vi "PosCtrl_Execute.vi"(5 "PosCtrl_Config_Params":T1={"Slope"=0.0, "Offset"=0.0, "Error Deadband"=0.0, "At Reference Count"=13, "Negate Output"=FALSE, "Max Allowd Position"=9e+30, "Min Allowd Position"=-9e+30}, 7 "MaxOutput":dbl, 8 "Rev Limit Switch":bool, 9 "Fwd Limit Switch":bool, 10 "CurrentPosition":dbl, 11 "TargetPosition":dbl) -> (1 "OnTarget":bool, 2 "PositionError":dbl, 3 "Output":dbl)   [LabVIEW 2019, in "Trajectory_Library.lvlib"]
doc: "This VI calculates closed loop position control output (CO), provided the Setpoint (SP), and Process Variable (PV). It incorporates a position deadband. It also incorporates output slowdown as the desired position is approached."
uses:
  TypeDef/PosCtrl_Tuning_Type.ctl
  Trajectory_Library.lvlib
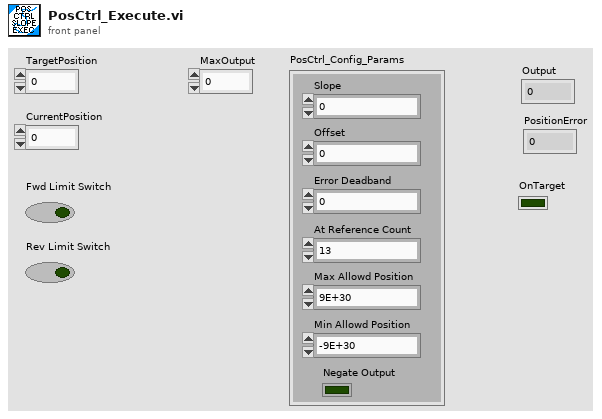
[diagram p1: front panel]
types:
  T1 = typedef "Trajectory_Library.lvlib/PosCtrl_Tuning_Type.ctl" = cluster{"Slope":dbl, "Offset":dbl, "Error Deadband":dbl, "At Reference Count":i32, "Negate Output":bool, "Max Allowd Position":dbl, "Min Allowd Position":dbl}
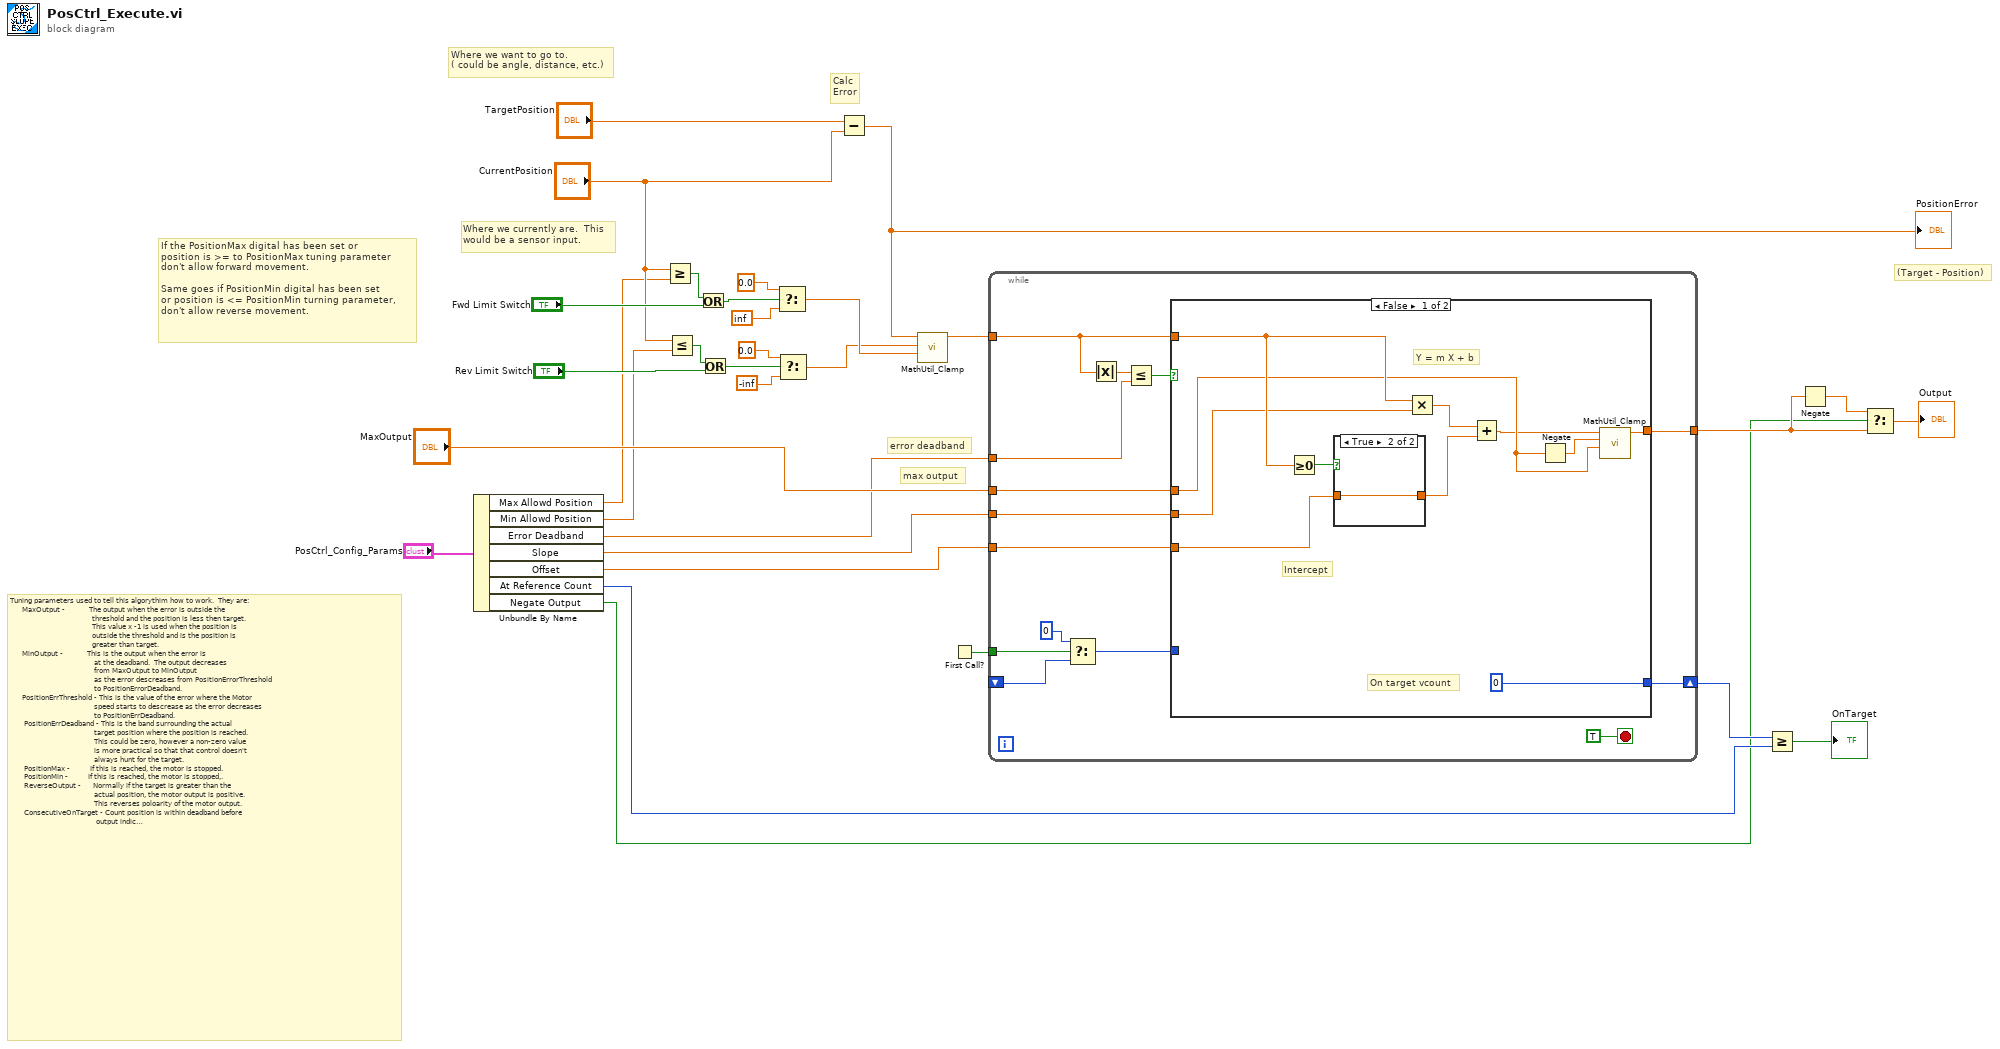
[diagram p0: block diagram]
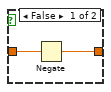
[diagram p2: hidden frame]
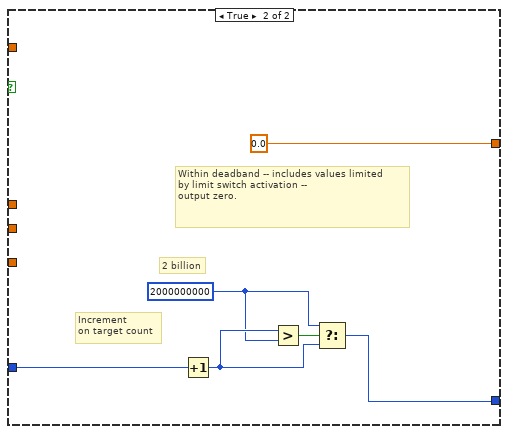
[diagram p3: hidden frame]
diagram:
  # "error deadband"
  # "max output"
  # "(Target - Position)"
  # "Calc\nError"
  # "If the PositionMax digital has been set or\nposition is >= to PositionMax tuning parameter\ndon't allow forward movement.\n\nSame goes if PositionMin digital has been set\nor position is <= PositionMin turning parameter, \ndon't allow reverse movement."
  # "Tuning parameters used to tell this algorythim how to work.  They are:\n      MaxOutput -            The output when the error is outside the \n                                         threshold and the position is less then target.\n                                         This value x -1 is used when the position is\n                                         outside the threshold and is the position is\n                                         greater than target.\n      MinOutput -            This is the output when the error is\n                                          at the deadband.  The output decreases\n                                          from MaxOutput to MinOutput\n                                          as the error descreases from PositionErrorThreshold\n                                          to PositionErrorDeadband.\n      PositionErrThreshold - This is the value of the error where the Motor\n                                          speed starts to descrease as the error decreases\n                                          to PositionErrDeadband.\n       PositionErrDeadband - This is the band surrounding the actual \n                                          target position where the position is reached.\n                                          This could be zero, however a non-zero value\n                                          is more practical so that that control doesn't\n                                          always hunt for the target.\n       PositionMax -          If this is reached, the motor is stopped.\n       PositionMin -          If this is reached, the motor is stopped,.\n       ReverseOutput -      Normally if the target is greater than the \n                                          actual position, the motor output is positive.\n                                          This reverses poloarity of the motor output.\n       ConsecutiveOnTarget - Count position is within deadband before\n                                           output indicates position goal has been\n                                           reached."
  # "Where we currently are.  This \nwould be a sensor input."
  # "Where we want to go to.\n( could be angle, distance, etc.)"
  n1 = Unbundle By Name("PosCtrl_Config_Params") -> ("Max Allowd Position"=w11:dbl, "Min Allowd Position"=w10:dbl, "Error Deadband"=w21:dbl, "Slope"=w20:dbl, "Offset"=w19:dbl, "At Reference Count"=w9:i32, "Negate Output"=w5:bool)
  n2 = Greater Or Equal?(x="CurrentPosition", y=w11) -> (x >= y?=w13:bool)
  n3 = Less Or Equal?(x="CurrentPosition", y=w10) -> (x <= y?=w14:bool)
  n4 = Or(x=w13, y="Fwd Limit Switch") -> (x .or. y?=w18:bool)
  n5 = Or(x=w14, y="Rev Limit Switch") -> (x .or. y?=w17:bool)
  n6 = Select(t=0.0, s=w18, f=inf) -> (s? t:f=w3:dbl)
  n7 = Select(t=0.0, s=w17, f=-inf) -> (s? t:f=w2:dbl)
  n8 = Subtract(x="TargetPosition", y="CurrentPosition") -> (x-y=w4:dbl)
  "PositionError" <- w4
  n9 = call "MathUtil_Clamp.vi"("High Limit"=w3, "Low Limit"=w2, "Value"=w4) -> ("Result"=w1:dbl)  [unwired: 8 in]
  n10 = First Call?() -> (First Call?: T/F=w26:bool)
  n11 = while {
    tunnel: w1 -> [w41]
    tunnel: w21 -> [w34]
    tunnel: [w42] -> w6
    tunnel: "MaxOutput" -> [w40]
    shift-right: [w39] -> w24
    shift-left: _ -> [w37]
    tunnel: w26 -> [w38]
    tunnel: w19 -> [w33]
    tunnel: w20 -> [w32]
    stop <- TRUE stop-if-true
    n12 = Select(t=0, s=w38, f=w37) -> (s? t:f=w36:i32)
    n13 = Absolute Value(x=w41) -> (abs(x)=w45:dbl)
    n14 = Less Or Equal?(x=w45, y=w34) -> (x <= y?=w43:bool)
    n15 = case shown="False" w43 {
      tunnel: [w46 0.0] -> w42
      tunnel: w41 -> [w56 _]
      tunnel: w40 -> [w48 _]
      tunnel: [0 w61] -> w39
      tunnel: w36 -> [_ w64]
      tunnel: w33 -> [w51 _]
      tunnel: w32 -> [w50 _]
      frame False {
        # "Y = m X + b"
        # "Intercept"
        # "On target vcount"
        n16 = Greater Or Equal To 0?(x=w56) -> (x >= 0?=w54:bool)
        n17 = case shown="True" w54 {
          tunnel: w51 -> [w58 w59]
          tunnel: [w57 w59] -> w52
          frame False {
            n18 = Negate(x=w58) -> (-x=w57:dbl)
          }
          frame True {
          }
        }
        n19 = Multiply(x=w56, y=w50) -> (x*y=w53:dbl)
        n20 = Add(x=w53, y=w52) -> (x+y=w47:dbl)
        n21 = Negate(x=w48) -> (-x=w49:dbl)
        n22 = call "MathUtil_Clamp.vi"("High Limit"=w48, "Low Limit"=w49, "Value"=w47) -> ("Result"=w46:dbl)  [unwired: 8 in]
      }
      frame True {
        w60 = 2000000000 ("y")
        # "2 billion"
        # "Increment\non target count"
        # "Within deadband -- includes values limited \nby limit switch activation --\noutput zero."
        n23 = Increment(x=w64) -> (x+1=w62:i32)
        n24 = Greater?(x=w62, y=w60) -> (0:w63:bool)
        n25 = Select(t=w60, s=w63, f=w62) -> (s? t:f=w61:i32)
      }
    }
  }
  n26 = Greater Or Equal?(x=w24, y=w9) -> (x >= y?=→"OnTarget":bool)
  n27 = Negate(x=w6) -> (-x=w7:dbl)
  n28 = Select(t=w7, s=w5, f=w6) -> (s? t:f=→"Output":dbl)
